vi "FunGen.vi"(4 "sampling info":cluster{"Fs":dbl, "#s":dbl}={"Fs"=100000000.0, "#s"=4000.0}, 5 "number of bits":i16=16, 6 "range (Vpp)":dbl=2.0, 7 "signal type":T1(ring), 8 "error in (no error)":errorcluster, 10 "amplitude":dbl=1.0 format="%0.2p", 11 "frequency":dbl=10.0 format="%0.2p") -> (0 "error out":errorcluster, 1 "Waveform Data":i16[](array[numeric]), 2 "Output Waveform Size":u32, 3 "Output Waveform (V)":waveform(dbl))   [LabVIEW 2020]
uses:
  <vilib>/measure/NI_MABase.lvlib
panel:
  out "Waveform Graph":waveform(dbl)(graph)
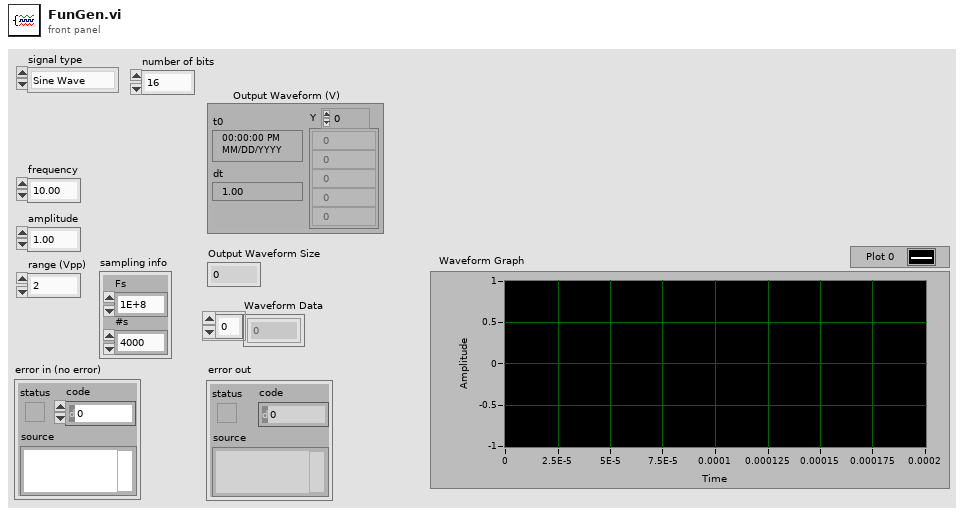
[diagram p1: front panel]
types:
  T1 = enum16{"Sine Wave", "Triangle Wave", "Square Wave", "Sawtooth Wave"}
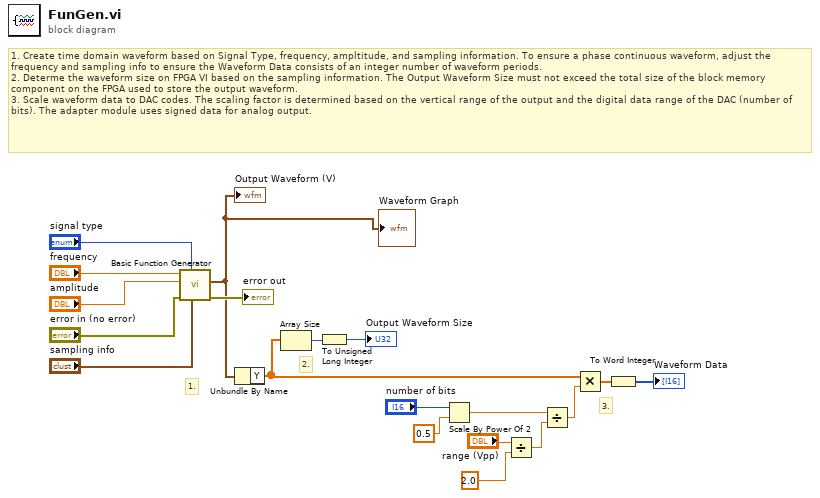
[diagram p0: block diagram]
diagram:
  # "2."
  # "1. Create time domain waveform based on Signal Type, frequency, ampltitude, and sampling information. To ensure a phase continuous waveform, adjust the frequency and sampling info to ensure the Waveform Data consists of an integer number of waveform periods.\n2. Determe the waveform size on FPGA VI based on the sampling information. The Output Waveform Size must not exceed the total size of the block memory component on the FPGA used to store the output waveform.\n3. Scale waveform data to DAC codes. The scaling factor is determined based on the vertical range of the output and the digital data range of the DAC (number of bits). The adapter module uses signed data for analog output."
  # "3."
  # "1."
  n1 = call <vilib>:"Basic Function Generator.vi"("sampling info"="sampling info", "signal type"="signal type", "error in (no error)"="error in (no error)", "amplitude"="amplitude", "frequency"="frequency") -> ("error out"=→"error out":errorcluster, "signal out"=w1:waveform(dbl))  [unwired: 4 in, 1 out]
  "Output Waveform (V)" <- w1
  "Waveform Graph" <- w1
  n2 = Unbundle By Name(w1) -> ("Y"=w13:dbl[])
  n3 = Array Size(array=w13) -> (size(s)=w19:i32)
  n4 = To Unsigned Long Integer(number=w19) -> (unsigned 32bit integer=→"Output Waveform Size":u32)
  n5 = Scale By Power Of 2(n="number of bits", x=0.5) -> (x*2^n=w14:dbl)
  n6 = Divide(x="range (Vpp)", y=2.0 ("x")) -> (x/y=w3:dbl)
  n7 = Divide(x=w14, y=w3) -> (x/y=w6:dbl)
  n8 = Multiply(x=w13, y=w6) -> (x*y=w17:dbl[])
  n9 = To Word Integer(number=w17) -> (16bit integer=→"Waveform Data":i16[])
